vi "Keithley 2450 Read Multiple.vi"(7 "Num Meas":u32=10, 8 "Compliance  Level (0.1)":dbl=0.1, 9 "Output Level (0)":dbl, 10 "Source Mode  (0: Voltage)":u16(ring) items=["Voltage", "Current"], 11 "VISA resource name":refnum<visa-resource-name>) -> (0 "Resistance":sgl[](array[numeric]), 1 "Current":sgl[](array[numeric]), 2 "Voltage":sgl[](array[numeric]))   [LabVIEW 2024]
doc: "This example shows how to configure a measurement and take multiple readings."
uses:
  Keithley/Keithley 2450/Keithley 2450.lvlib
  Keithley/archive/Keithley 24XX/Keithley 24XX.lvlib
panel:
  out "error out":errorcluster
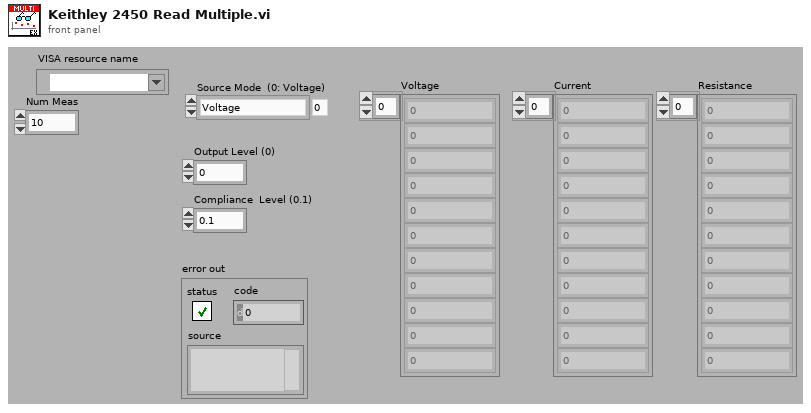
[diagram p1: front panel]
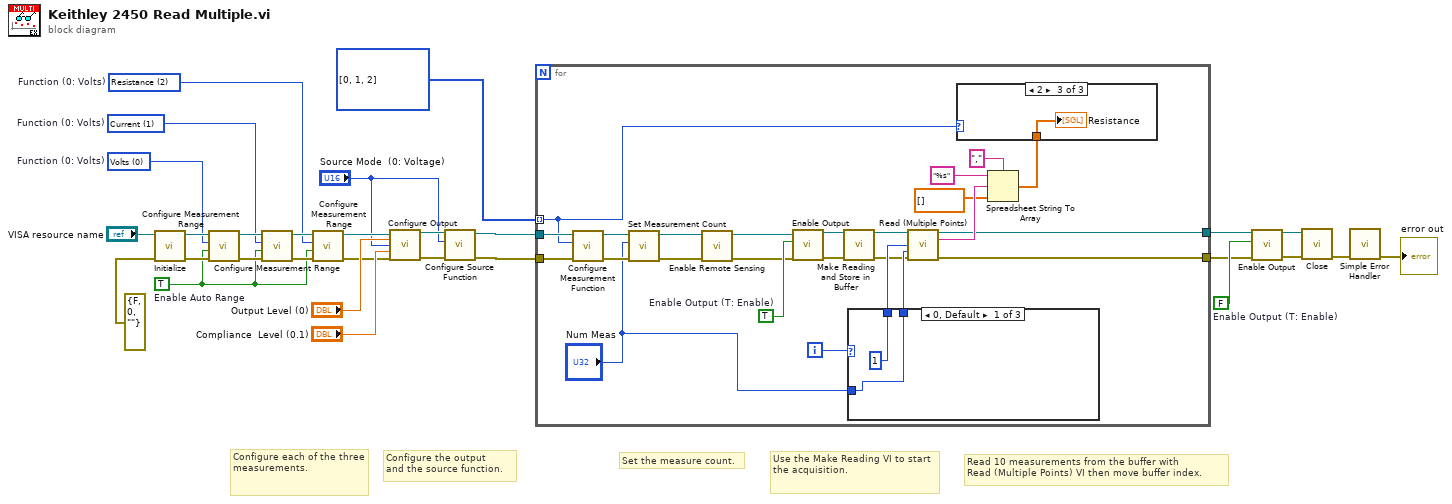
[diagram p0: block diagram]
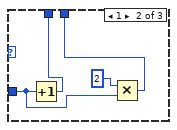
[diagram p2: hidden frame]
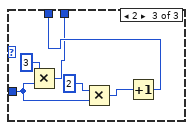
[diagram p3: hidden frame]
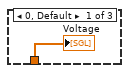
[diagram p4: hidden frame]
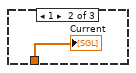
[diagram p5: hidden frame]
diagram:
  w8 = u16[] [0, 1, 2] items=["Volts", "Current", "Resistance"]
  w13 = FALSE  # Enable Output (T: Enable)
  w18 = u16 2 items=["Volts", "Current", "Resistance"]  # Function (0: Volts)
  w19 = u16 1 items=["Volts", "Current", "Resistance"]  # Function (0: Volts)
  w20 = u16 0 items=["Volts", "Current", "Resistance"]  # Function (0: Volts)
  w21 = TRUE  # Enable Auto Range
  # "Read 10 measurements from the buffer with \nRead (Multiple Points) VI then move buffer index."
  # "Set the measure count."
  # "Use the Make Reading VI to start the acquisition."
  # "Configure the output \nand the source function."
  # "Configure each of the three measurements."
  n1 = call "Initialize.vi"("error in (no error)"=errorcluster {"status"=FALSE, "code"=0, "source"=""}, "VISA resource name"="VISA resource name") -> ("error out"=w26:errorcluster, "VISA resource name out"=w27:refnum<visa-resource-name>)  [unwired: 8 in]
  n2 = call "Configure Measurement Range.vi"("error in (no error)"=w26, "Enable Auto Range (T:Enable)"=w21, "Function (0: Volts)"=w20, "VISA resource name"=w27) -> ("error out"=w25:errorcluster, "VISA resource name out"=w24:refnum<visa-resource-name>)  [unwired: 6 in]
  n3 = call "Configure Measurement Range.vi"("error in (no error)"=w25, "Enable Auto Range (T:Enable)"=w21, "Function (0: Volts)"=w19, "VISA resource name"=w24) -> ("error out"=w22:errorcluster, "VISA resource name out"=w23:refnum<visa-resource-name>)  [unwired: 6 in]
  n4 = call "Configure Measurement Range.vi"("error in (no error)"=w22, "Enable Auto Range (T:Enable)"=w21, "Function (0: Volts)"=w18, "VISA resource name"=w23) -> ("error out"=w11:errorcluster, "VISA resource name out"=w12:refnum<visa-resource-name>)  [unwired: 6 in]
  n5 = call "Configure Output.vi"("VISA resource name"=w12, "Source Level (0)"="Output Level (0)", "Source Mode  (0: Voltage)"="Source Mode  (0: Voltage)", "Source Limit Level (0.1)"="Compliance  Level (0.1)", "error in (no error)"=w11) -> ("VISA resource name out"=w6:refnum<visa-resource-name>, "error out"=w7:errorcluster)  [unwired: 9 in]
  n6 = call "Configure Source Function.vi"("error in (no error)"=w7, "Function (0: Volts)"="Source Mode  (0: Voltage)", "VISA resource name"=w6) -> ("error out"=w4:errorcluster, "VISA resource name out"=w5:refnum<visa-resource-name>)  [unwired: 7 in]
  n7 = for {
    tunnel: [w44] -> w10
    tunnel: [w43] -> w9
    tunnel: w4 -> [w54]
    tunnel: w5 -> [w53]
    tunnel: w8 -> [w52] mode=indexing
    i -> [w40]
    w37 = TRUE  # Enable Output (T: Enable)
    n8 = call "Configure Measurement Function.vi"("error in (no error)"=w54, "Function (0: Volts)"=w52, "VISA resource name"=w53) -> ("error out"=w51:errorcluster, "VISA resource name out"=w50:refnum<visa-resource-name>)  [unwired: 7 in]
    n9 = call "Set Measurement Count.vi"("error in (no error)"=w51, "Measurement Count"="Num Meas", "VISA resource name"=w50) -> ("error out"=w32:errorcluster, "VISA resource name out"=w34:refnum<visa-resource-name>)  [unwired: 7 in]
    n10 = call "Enable Remote Sensing.vi"("error in (no error)"=w32, "VISA resource name"=w34) -> ("error out"=w31:errorcluster, "VISA resource name out"=w33:refnum<visa-resource-name>)  [unwired: 8 in]
    n11 = call "Enable Output.vi"("error in (no error)"=w31, "Enable Output (T: Enable)"=w37, "VISA resource name"=w33) -> ("error out"=w35:errorcluster, "VISA resource name out"=w36:refnum<visa-resource-name>)  [unwired: 7 in]
    n12 = call "Make Reading and Store in Buffer.vi"("VISA resource name"=w36, "error in (no error)"=w35) -> ("VISA resource name out"=w39:refnum<visa-resource-name>, "error out"=w38:errorcluster)  [unwired: 12 in]
    n13 = case shown="0, Default" w40 {
      tunnel: [u32 1 ("millisecond multiple") w60 w64] -> w42
      tunnel: [w55 w57 w61] -> w41
      tunnel: "Num Meas" -> [w55 w58 w62]
      frame 0, Default {
      }
      frame 1 {
        n14 = Increment(x=w58) -> (x+1=w60:u32)
        n15 = Multiply(x=u32 2 ("millisecond multiple"), y=w58) -> (x*y=w57:u32)
      }
      frame 2 {
        n16 = Multiply(x=u32 3 ("millisecond multiple"), y=w62) -> (x*y=w61:u32)
        n17 = Multiply(x=u32 2 ("millisecond multiple"), y=w62) -> (x*y=w65:u32)
        n18 = Increment(x=w65) -> (x+1=w64:u32)
      }
    }
    n19 = call "Read (Multiple Points).vi"("VISA resource name"=w39, "Start Index (1)"=w42, "End Index (1)"=w41, "error in (no error)"=w38) -> ("VISA resource name out"=w44:refnum<visa-resource-name>, "Data out"=w49:string, "error out"=w43:errorcluster)  [unwired: 9 in]
    n20 = Spreadsheet String To Array(delimiter (Tab)=",", format string="%s", spreadsheet string=w49, array type (2D Dbl)=dbl[] []) -> (array=w48:dbl[])
    n21 = case shown="2" w52 {
      tunnel: w48 -> [w67 w68 w69]
      frame 0, Default {
        "Voltage" <- w67
      }
      frame 1 {
        "Current" <- w68
      }
      frame 2 {
        "Resistance" <- w69
      }
    }
  }
  n22 = call "Enable Output.vi"("error in (no error)"=w9, "Enable Output (T: Enable)"=w13, "VISA resource name"=w10) -> ("error out"=w14:errorcluster, "VISA resource name out"=w15:refnum<visa-resource-name>)  [unwired: 7 in]
  n23 = call "Close.vi"("error in (no error)"=w14, "VISA resource name"=w15) -> ("error out"=w29:errorcluster)  [unwired: 9 in]
  n24 = call <vilib>:"Simple Error Handler.vi"("error in (no error)"=w29) -> ("error out"=→"error out":errorcluster)  [unwired: 4 in, 4 out]
